vi "DAC Run.vi"(8 "error in":errorcluster, 11 "DAC FTCU in":refnum<class "DAC FTCU.lvclass">) -> (0 "error out":errorcluster, 3 "DAC FTCU out":refnum<class "DAC FTCU.lvclass">)   [LabVIEW 2019, in "DAC.lvlib" / "DAC FTCU.lvclass"]
uses:
  DAC FTCU.lvclass
  C:/Users/wg/Documents/LV_Projects/test-stand/App/DAC/DAC.lvclass
  DAC.lvclass/DAC.ctl
  DAC.lvclass
  Results/Results Method.ctl
  Results/Results.lvlib
  Results/DeepU Results/DeepU Results.lvclass
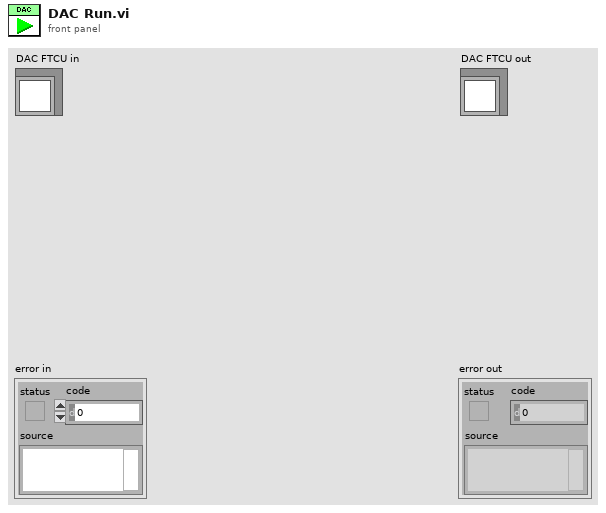
[diagram p1: front panel]
types:
  T1 = typedef "Results.lvlib/Results Method.ctl" = enum16{"Get", "Set"}
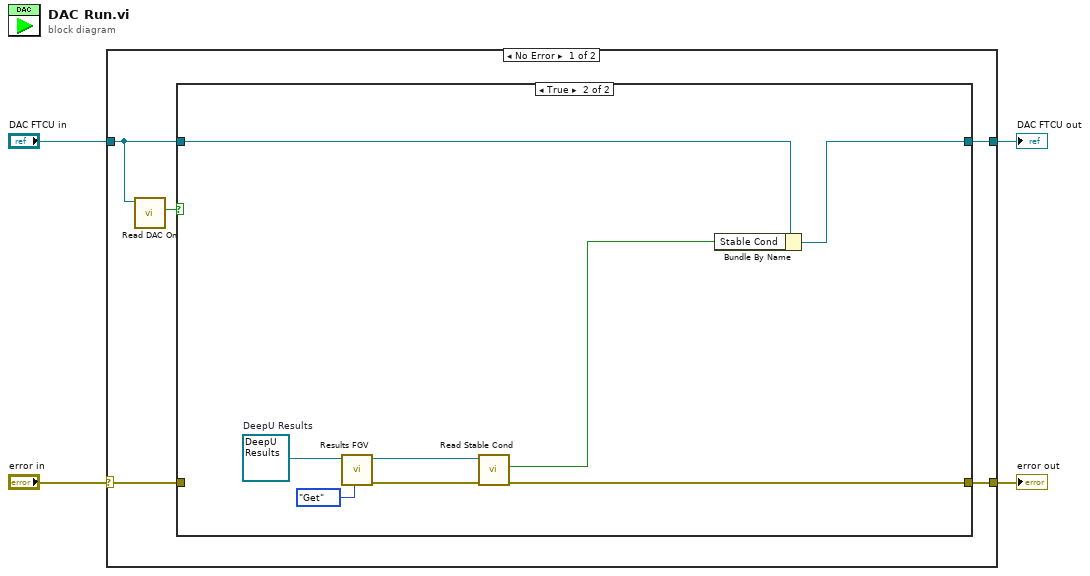
[diagram p0: block diagram]
diagram:
  n1 = case shown="No Error" "error in" {
    selector: "error in" -> [w7 w21]
    tunnel: [w6 w21] -> w2
    tunnel: [w8 w20] -> w1
    tunnel: "DAC FTCU in" -> [w5 w20]
    frame No Error {
      n2 = call "Read DAC On.vi"("DAC in"=w5) -> ("DAC On"=w9:bool)  [unwired: 8 in, 2 out]
      n3 = case shown="True" w9 {
        tunnel: w5 -> [w11 w17]
        tunnel: [w11 w16] -> w8
        tunnel: w7 -> [w10 _]
        tunnel: [w10 w12] -> w6
        frame False {
        }
        frame True {
          w19 = refnum<class "DeepU Results.lvclass"> refnum  # DeepU Results
          n4 = call-dynamic "Results FGV.vi"("Method"=Results_Method."Get", "DeepU Results in"=w19) -> ("error out"=w13:errorcluster, "DeepU Results out"=w15:refnum<class "DeepU Results.lvclass">)  [unwired: 8 in]
          n5 = call "Read Stable Cond.vi"("error in (no error)"=w13, "DeepU Results in"=w15) -> ("error out"=w12:errorcluster, "Stable Cond"=w14:bool)  [unwired: 7 in, 1 out]
          n6 = Bundle By Name(cluster=w17, "Stable Cond"=w14) -> (w16:refnum<class "DAC FTCU.lvclass">)
        }
      }
    }
    frame Error {
    }
  }
  "error out" <- w2
  "DAC FTCU out" <- w1
